vi "Decimate Waveforms.vi"(8 "error in (no error)":errorcluster, 10 "Decimation":i32, 11 "Waveforms in":waveform(dbl)[](array[waveform])) -> (0 "error out":errorcluster, 3 "Waveforms out":waveform(dbl)[](array[waveform]))   [LabVIEW 2019, in "DSP.lvclass"]
uses:
  <vilib>/Analysis/2dsp.llb/Decimate (single shot, DBL).vi
  DSP.lvclass
  <vilib>/Analysis/NI_AALPro.lvlib
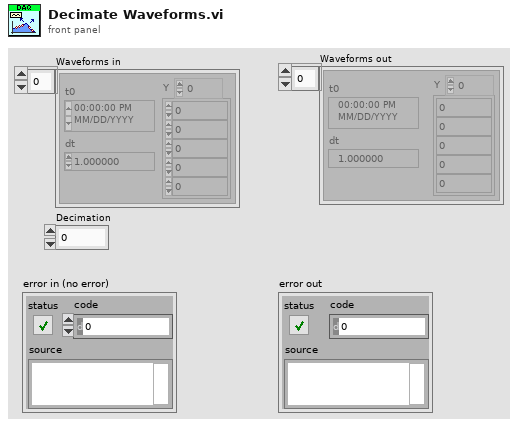
[diagram p1: front panel]
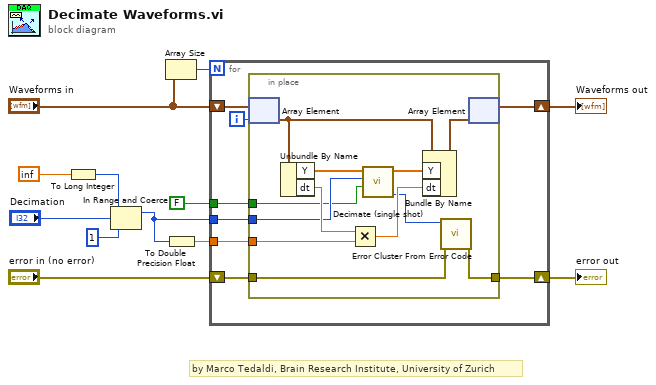
[diagram p0: block diagram]
diagram:
  # "by Marco Tedaldi, Brain Research Institute, University of Zurich"
  n1 = To Long Integer(number=inf) -> (32bit integer=w2:i32)
  n2 = In Range and Coerce(upper limit=w2, x="Decimation", lower limit=1) -> (coerced(x)=w5:i32)  [unwired: 1 out]
  n3 = Array Size(array="Waveforms in") -> (size(s)=w12:i32)
  n4 = To Double Precision Float(number=w5) -> (double precision float=w6:dbl)
  n5 = for {
    N: w12 -> [_]
    tunnel: w6 -> [w20]
    tunnel: w5 -> [w19]
    tunnel: FALSE ("averaging") -> [w18]
    shift-right: [w14] -> w8
    shift-left: "Waveforms in" -> [w16]
    shift-right: [w17] -> w10
    shift-left: "error in (no error)" -> [w13]
    i -> [w15]
    n6 = in-place {
      in-place-border: w20 -> [w30]
      in-place-border: w19 -> [w29]
      in-place-border: w18 -> [w27]
      in-place-border: [w24] -> w17
      in-place-border: w13 -> [w25]
      n7 = in-place-array #1(w16, w15) -> (w22:waveform(dbl))
      n8 = Unbundle By Name(w22) -> ("Y"=w23:dbl[], "dt"=w31:dbl)
      n9 = Multiply(x=w31, y=w30) -> (x*y=w28:dbl)
      n10 = call-poly <vilib>:"Decimate (single shot).vi"("averaging"=w27, "decimating factor"=w29, "X"=w23) -> ("error"=w26:i32, "Decimated Array"=w32:dbl[])  [unwired: 7 in]
      n11 = Bundle By Name(cluster=w22, "Y"=w32, "dt"=w28) -> (w21:waveform(dbl))
      n12 = call <vilib>:"Error Cluster From Error Code.vi"("error in (no error)"=w25, "error code (0)"=w26) -> ("error out"=w24:errorcluster)  [unwired: 7 in]
      n13 = in-place-array #1(w21) -> (w14:waveform(dbl)[])  [unwired: 1 out]
    }
  }
  "error out" <- w10
  "Waveforms out" <- w8
